vi "CII.vi"(0 "Wheel":dbl, 1 "Throttle":dbl) -> (7 "RightDrive":dbl, 8 "LeftDrive":dbl)   [LabVIEW 2015]
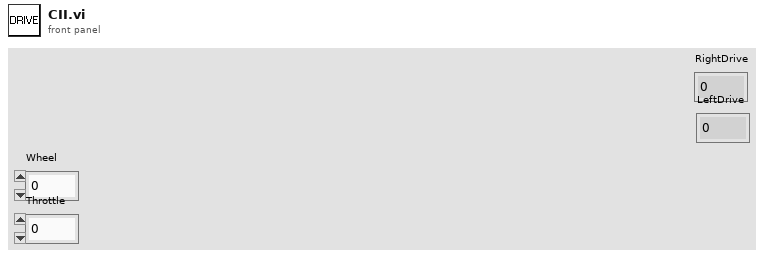
[diagram p1: front panel]
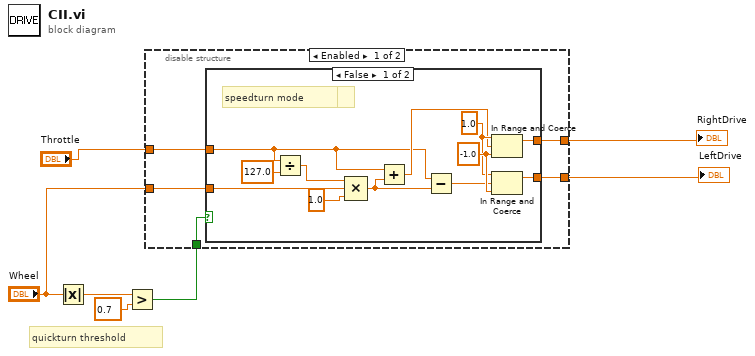
[diagram p0: block diagram]
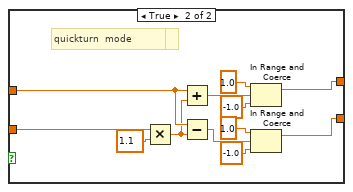
[diagram p2: hidden frame]
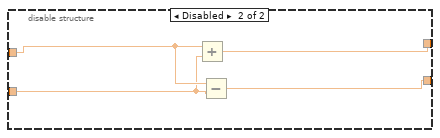
[diagram p3: hidden frame]
diagram:
  # "quickturn threshold"
  n1 = Absolute Value(x="Wheel") -> (abs(x)=w7:dbl)
  n2 = Greater?(x=w7, y=0.7) -> (0:w6:bool)
  n3 = disable-structure shown="Enabled" {
    disable-tunnel: w6 -> [w12 _]
    disable-tunnel: [w11 w38] -> w4
    disable-tunnel: [w10 w37] -> w3
    disable-tunnel: "Throttle" -> [w9 w40]
    disable-tunnel: "Wheel" -> [w8 w39]
    frame Enabled {
      n4 = case shown="False" w12 {
        tunnel: w9 -> [w13 w34]
        tunnel: w8 -> [w16 w36]
        tunnel: [w20 w27] -> w11
        tunnel: [w19 w30] -> w10
        frame False {
          w18 = -1.0 ("upper limit")
          w17 = 1.0 ("milliseconds to wait")
          # "speedturn constant"
          # "speedturn mode"
          n5 = Divide(x=w13, y=127.0) -> (x/y=w23:dbl)
          n6 = Compound Arithmetic op=MULTIPLY(w23, w16, 1.0) -> (w21:dbl)
          n7 = Add(x=w13, y=w21) -> (x+y=w14:dbl)
          n8 = Subtract(x=w13, y=w21) -> (x-y=w15:dbl)
          n9 = In Range and Coerce(upper limit=w17, x=w14, lower limit=w18) -> (coerced(x)=w20:dbl)  [unwired: 1 out]
          n10 = In Range and Coerce(upper limit=w17, x=w15, lower limit=w18) -> (coerced(x)=w19:dbl)  [unwired: 1 out]
        }
        frame True {
          # "quickturn constant"
          # "quickturn  mode"
          n11 = Multiply(x=w36, y=1.1) -> (x*y=w33:dbl)
          n12 = Add(x=w34, y=w33) -> (x+y=w26:dbl)
          n13 = Subtract(x=w34, y=w33) -> (x-y=w25:dbl)
          n14 = In Range and Coerce(upper limit=1.0, x=w26, lower limit=-1.0) -> (coerced(x)=w27:dbl)  [unwired: 1 out]
          n15 = In Range and Coerce(upper limit=1.0, x=w25, lower limit=-1.0 ("upper limit")) -> (coerced(x)=w30:dbl)  [unwired: 1 out]
        }
      }
    }
    frame Disabled {
      n16 = Add(x=w40, y=w39) -> (x+y=w38:dbl)
      n17 = Subtract(x=w40, y=w39) -> (x-y=w37:dbl)
    }
  }
  "RightDrive" <- w4
  "LeftDrive" <- w3
